vi "PN_P.vi"() -> ()   [LabVIEW 2020]
panel:
  out "PN":string
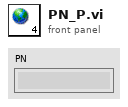
[diagram p1: front panel]
diagram:
